vi "CODMn流程.vi"   [LabVIEW 2016]
types:
  T1 = enum16{"步骤1", "步骤2", "步骤3", "步骤4", "步骤5", "步骤6", "步骤7", "步骤8", "步骤9", "步骤10"}
  T2 = enum32{"Bad", "Idle", "Run top level", "Running"}
  T3 = cluster{"系统时间":timestamp, "工作状态":u16, "测量模式":u16, "告警代码":enum16{"无告警", "缺试剂告警", "缺水样告警", "缺蒸馏水告警", "缺标液告警", "仪表漏液告警", "标定异常告警", "超量程告警", "加热异常", "低试剂预警", "超上限告警", "超下限告警", "仪表内部其他异常", "滴定异常告警", "电极异常告警", "量程切换告警", "参数设置告警", "PH电极电位异常", "电导率电极异常", "浊度光度异常", "溶解氧电极异常", "溶解氧光强异常", "温度异常告警", "PH异常告警", "溶解氧异常告警", "电导率异常告警", "浊度异常告警", "叶绿素异常告警", "藻密度异常告警", "蓝绿藻异常告警", "ORP异常告警", "氨氮异常告警", "清洁刷异常告警", "SD卡异常告警", "蓝牙异常告警", "Wifi异常告警", "流程异常告警"}, "故障代码":enum16{"无故障", "电机故障", "温度故障", "通讯故障", "滴定故障"}, "日志代码":u16, "软件版本":u16, "F0":sgl, "F1":sgl, "F2":sgl, "F3":sgl, "T":sgl, "H":sgl, "id":u16, "flowid":u16, "量程":u16}
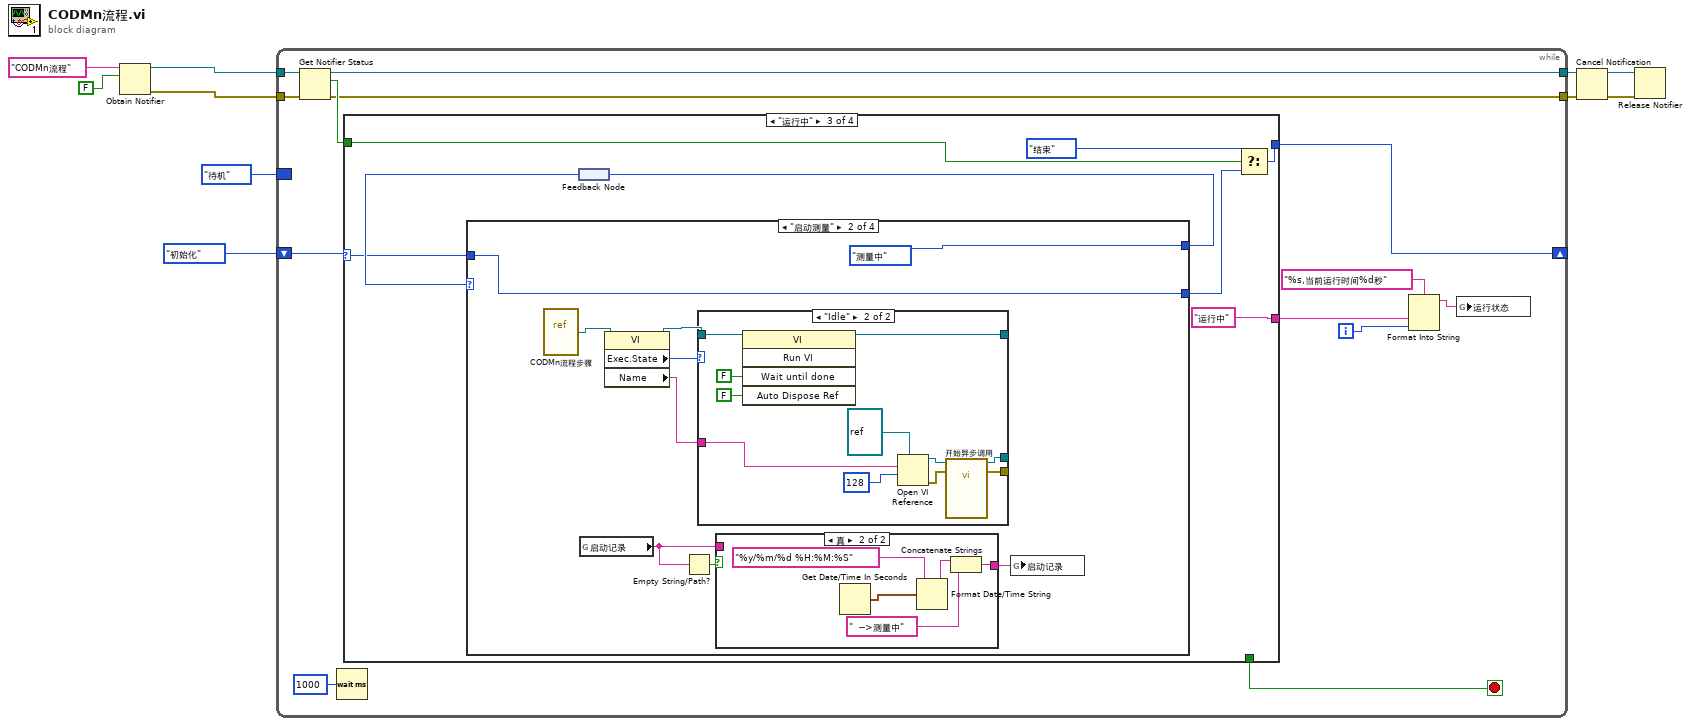
[diagram p0: block diagram]
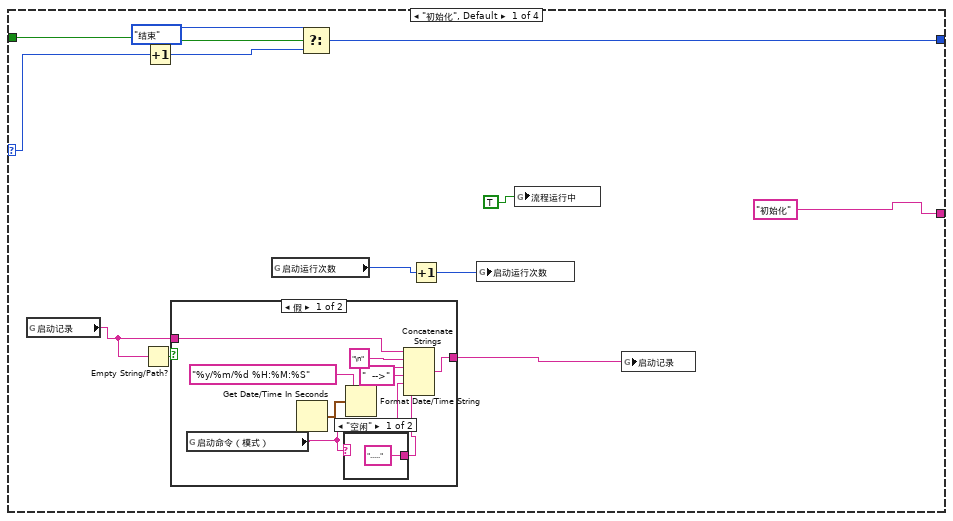
[diagram p2: hidden frame]
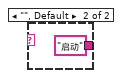
[diagram p3: hidden frame]
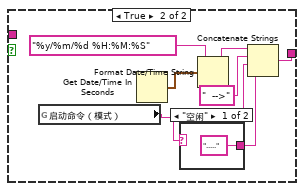
[diagram p4: hidden frame]
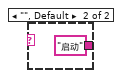
[diagram p5: hidden frame]
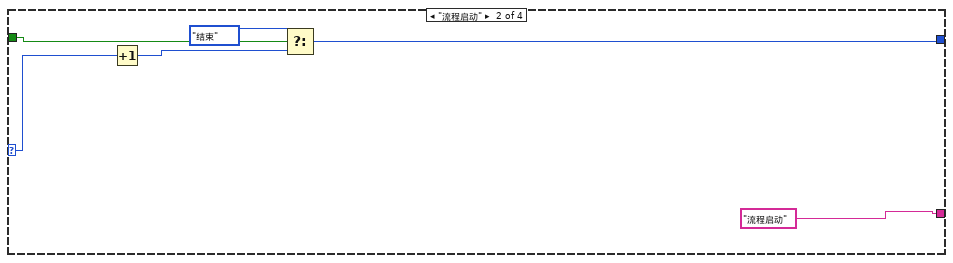
[diagram p6: hidden frame]
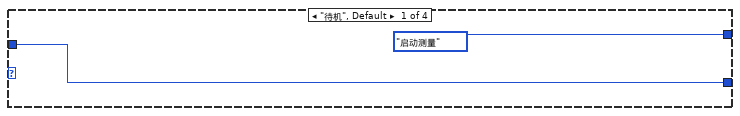
[diagram p7: hidden frame]
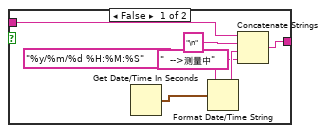
[diagram p8: hidden frame]
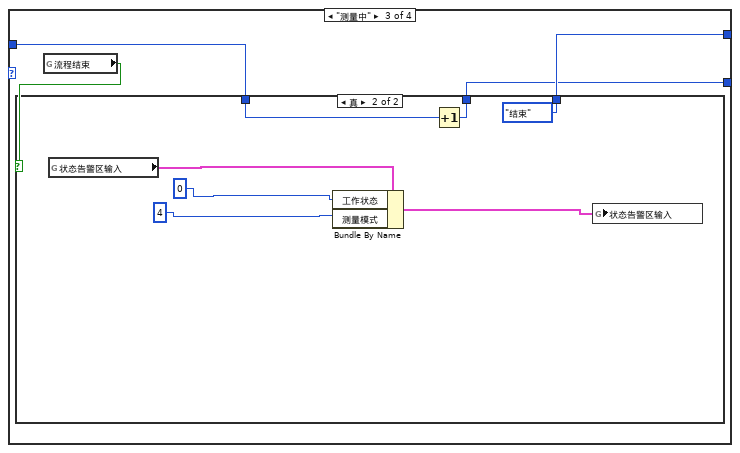
[diagram p10: hidden frame]
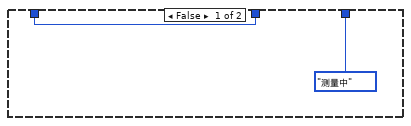
[diagram p11: hidden frame]
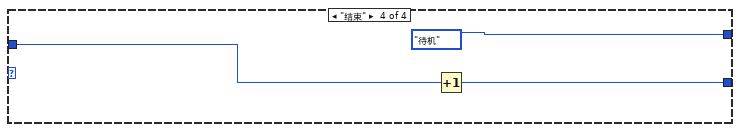
[diagram p12: hidden frame]
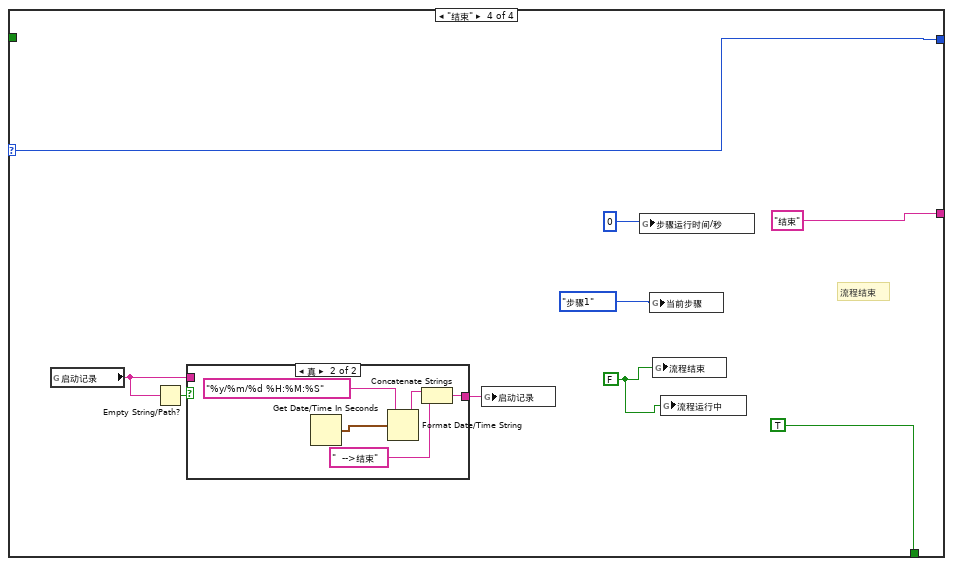
[diagram p13: hidden frame]
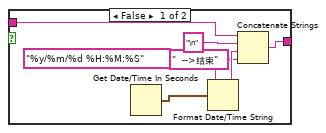
[diagram p14: hidden frame]
diagram:
  n1 = Obtain Notifier(name (unnamed)="CODMn流程" ("名称（未命名）"), notification data type=FALSE) -> (notifier out=w7:refnum<notifier>, error out=w6:errorcluster)  [unwired: 2 in, 1 out]
  n2 = while {
    shift-right: [w20] -> _
    shift-left: enum16{"初始化", "流程启动", "运行中", "结束"}."初始化" ("枚举") -> [w23]
    tunnel: w7 -> [w15]
    tunnel: w6 -> [w14]
    tunnel: [w13] -> w5
    tunnel: [w12] -> w4
    border: enum16{"待机", "启动测量", "测量中", "结束"}."待机" -> [_]
    i -> [w18]
    stop <- w16 stop-if-true
    n3 = Get Notifier Status(notifier=w15, error in (no error)=w14) -> (notifier out=w13:refnum<notifier>, current notification=w21:bool, error out=w12:errorcluster)  [unwired: 2 out]
    n4 = Wait (ms)(milliseconds to wait=u32 1000 ("等待时间（毫秒）")) -> ()  [unwired: 1 out]
    n5 = case shown="\"运行中\"" w23 {
      selector: w23 -> [w33 w58 w64 w127]
      tunnel: [_ _ _ TRUE ("x")] -> w16
      tunnel: w21 -> [w35 w59 w68 _]
      tunnel: [w31 w57 w63 w127] -> w20
      tunnel: ["初始化" ("输入 1") "流程启动" ("输入 1") "运行中" ("输入 1") "结束" ("输入 1")] -> w17
      frame "初始化", Default {
        n6 = global read "CODMn全局.vi" "启动记录"() -> (w24:string)
        n7 = Empty String/Path?(string/path=w24) -> (empty?=w29:bool)
        n8 = Increment(x=w33) -> (x+1=w32:enum16{"初始化", "流程启动", "运行中", "结束"})
        n9 = case shown="假" w29 {
          tunnel: w24 -> [w44 _]
          tunnel: [w39 w50] -> w25
          frame False {
            n10 = global read "CODMn全局.vi" "启动命令（模式）"() -> (w37:string)
            n11 = Get Date/Time In Seconds() -> (seconds since 1Jan1904=w42:timestamp)
            n12 = case shown="\"空闲\"" w37 {
              tunnel: ["....." ("字符串") "启动" ("字符串")] -> w36
              frame "空闲" {
              }
              frame "", Default {
              }
            }
            n13 = Format Date/Time String(time format string (%c)="%y/%m/%d %H:%M:%S" ("时间格式字符串(%c)"), seconds (now)=w42) -> (date/time string=w40:string)  [unwired: 1 in]
            n14 = Concatenate Strings(w44, "\n" ("字符串"), w40, "  -->" ("字符串"), w37, w36) -> (w39:string)
          }
          frame True {
            n15 = global read "CODMn全局.vi" "启动命令（模式）"() -> (w48:string)
            n16 = Get Date/Time In Seconds() -> (seconds since 1Jan1904=w53:timestamp)
            n17 = case shown="\"空闲\"" w48 {
              tunnel: ["....." ("字符串") "启动" ("字符串")] -> w47
              frame "空闲" {
              }
              frame "", Default {
              }
            }
            n18 = Format Date/Time String(time format string (%c)="%y/%m/%d %H:%M:%S" ("时间格式字符串(%c)"), seconds (now)=w53) -> (date/time string=w51:string)  [unwired: 1 in]
            n19 = Concatenate Strings(w51, "  -->" ("字符串"), w48, w47) -> (w50:string)
          }
        }
        n20 = global read "CODMn全局.vi" "启动运行次数"() -> (w27:i32)
        n21 = Select(t=enum16{"初始化", "流程启动", "运行中", "结束"}."结束" ("枚举"), s=w35, f=w32) -> (s? t:f=w31:enum16{"初始化", "流程启动", "运行中", "结束"})
        n22 = Increment(x=w27) -> (x+1=w26:i32)
        n23 = global write "CODMn全局.vi" "启动运行次数"(w26) -> ()
        n24 = global write "CODMn全局.vi" "流程运行中"(TRUE ("流程运行中")) -> ()
        n25 = global write "CODMn全局.vi" "启动记录"(w25) -> ()
      }
      frame "流程启动" {
        n26 = Increment(x=w58) -> (x+1=w60:enum16{"初始化", "流程启动", "运行中", "结束"})
        n27 = Select(t=enum16{"初始化", "流程启动", "运行中", "结束"}."结束" ("枚举"), s=w59, f=w60) -> (s? t:f=w57:enum16{"初始化", "流程启动", "运行中", "结束"})
      }
      frame "运行中" {
        n28 = feedback #1() -> (w67:enum16{"待机", "启动测量", "测量中", "结束"})
        n29 = case shown="\"启动测量\"" w67 {
          tunnel: [enum16{"待机", "启动测量", "测量中", "结束"}."启动测量" enum16{"待机", "启动测量", "测量中", "结束"}."测量中" w108 enum16{"待机", "启动测量", "测量中", "结束"}."待机"] -> w66
          tunnel: [w70 w79 w106 w119] -> w65
          tunnel: w64 -> [w70 w79 w107 w118]
          frame "待机", Default {
          }
          frame "启动测量" {
            n30 = vi-ref "CODMn流程步骤.vi"() -> (w75:refnum<vi>)
            n31 = global read "CODMn全局.vi" "启动记录"() -> (w73:string)
            n32 = property class="VI"(reference=w75) -> (reference out=w76:refnum<vi>, "Exec.State"=w77:T2, "Name"=w78:string)  [unwired: 1 in, 1 out]
            n33 = Empty String/Path?(string/path=w73) -> (empty?=w74:bool)
            n34 = case shown="\"Idle\"" w77 {
              tunnel: w76 -> [w93 w101]
              tunnel: [w93 w102] -> _
              tunnel: w78 -> [_ w100]
              tunnel: [_ w95] -> _
              tunnel: [_ w94] -> _
              frame "Bad", Default {
              }
              frame "Idle" {
                n35 = invoke class="VI" method="Run VI"(reference=w101, "Wait until done"=FALSE ("结束前等待"), "Auto Dispose Ref"=FALSE ("自动销毁引用")) -> (reference out=w102:refnum<vi>)  [unwired: 2 in, 4 out]
                n36 = Open VI Reference(type specifier VI Refnum (for type only)=refnum<vi> refnum ("类型说明符VI引用句柄（仅用于类型）"), vi path=w100, options=128 ("选项")) -> (vi reference=w96:refnum<vi>, error out=w98:errorcluster)  [unwired: 3 in]
                n37 = call-by-ref "开始异步调用"(reference=w96, error in=w98) -> (reference out=w95:refnum<vi>, error out=w94:errorcluster)  [unwired: 12 in]
              }
            }
            n38 = case shown="真" w74 {
              tunnel: w73 -> [w87 _]
              tunnel: [w81 w88] -> w72
              frame False {
                n39 = Get Date/Time In Seconds() -> (seconds since 1Jan1904=w85:timestamp)
                n40 = Format Date/Time String(time format string (%c)="%y/%m/%d %H:%M:%S" ("时间格式字符串(%c)"), seconds (now)=w85) -> (date/time string=w83:string)  [unwired: 1 in]
                n41 = Concatenate Strings(w87, "\n" ("字符串"), w83, "  -->测量中" ("字符串")) -> (w81:string)
              }
              frame True {
                n42 = Get Date/Time In Seconds() -> (seconds since 1Jan1904=w92:timestamp)
                n43 = Format Date/Time String(time format string (%c)="%y/%m/%d %H:%M:%S" ("时间格式字符串(%c)"), seconds (now)=w92) -> (date/time string=w90:string)  [unwired: 1 in]
                n44 = Concatenate Strings(w90, "  -->测量中" ("字符串")) -> (w88:string)
              }
            }
            n45 = global write "CODMn全局.vi" "启动记录"(w72) -> ()
          }
          frame "测量中" {
            n46 = global read "CODMn全局.vi" "流程结束"() -> (w105:bool)
            n47 = case shown="真" w105 {
              tunnel: [enum16{"待机", "启动测量", "测量中", "结束"}."测量中" enum16{"待机", "启动测量", "测量中", "结束"}."结束"] -> w108
              tunnel: w107 -> [w109 w116]
              tunnel: [w109 w115] -> w106
              frame False {
              }
              frame True {
                n48 = global read "CODMn全局.vi" "状态告警区输入"() -> (w112:T3)
                n49 = Bundle By Name(cluster=w112, "工作状态"=u16 0, "测量模式"=u16 4) -> (w111:T3)
                n50 = Increment(x=w116) -> (x+1=w115:enum16{"初始化", "流程启动", "运行中", "结束"})
                n51 = global write "CODMn全局.vi" "状态告警区输入"(w111) -> ()
              }
            }
          }
          frame "结束" {
            n52 = Increment(x=w118) -> (x+1=w119:enum16{"初始化", "流程启动", "运行中", "结束"})
          }
        }
        n53 = feedback-in #1(w66) -> ()
        n54 = Select(t=enum16{"初始化", "流程启动", "运行中", "结束"}."结束" ("枚举"), s=w68, f=w65) -> (s? t:f=w63:enum16{"初始化", "流程启动", "运行中", "结束"})
      }
      frame "结束" {
        w121 = FALSE ("流程结束")
        # "流程结束"
        n55 = global read "CODMn全局.vi" "启动记录"() -> (w125:string)
        n56 = Empty String/Path?(string/path=w125) -> (empty?=w126:bool)
        n57 = case shown="真" w126 {
          tunnel: w125 -> [w136 _]
          tunnel: [w130 w137] -> w122
          frame False {
            n58 = Get Date/Time In Seconds() -> (seconds since 1Jan1904=w134:timestamp)
            n59 = Format Date/Time String(time format string (%c)="%y/%m/%d %H:%M:%S" ("时间格式字符串(%c)"), seconds (now)=w134) -> (date/time string=w132:string)  [unwired: 1 in]
            n60 = Concatenate Strings(w136, "\n" ("字符串"), w132, "  -->结束" ("字符串")) -> (w130:string)
          }
          frame True {
            n61 = Get Date/Time In Seconds() -> (seconds since 1Jan1904=w141:timestamp)
            n62 = Format Date/Time String(time format string (%c)="%y/%m/%d %H:%M:%S" ("时间格式字符串(%c)"), seconds (now)=w141) -> (date/time string=w139:string)  [unwired: 1 in]
            n63 = Concatenate Strings(w139, "  -->结束" ("字符串")) -> (w137:string)
          }
        }
        n64 = global write "CODMn全局.vi" "启动记录"(w122) -> ()
        n65 = global write "CODMn全局.vi" "步骤运行时间/秒"(0 ("运行时间/秒")) -> ()
        n66 = global write "CODMn全局.vi" "当前步骤"(T1."步骤1" ("当前步骤 2")) -> ()
        n67 = global write "CODMn全局.vi" "流程结束"(w121) -> ()
        n68 = global write "CODMn全局.vi" "流程运行中"(w121) -> ()
      }
    }
    n69 = Format Into String(format string="%s,当前运行时间%d秒" ("格式字符串"), w17, w18) -> (resulting string=w11:string)  [unwired: 2 in, 1 out]
    n70 = global write "CODMn全局.vi" "运行状态"(w11) -> ()
  }
  n71 = Cancel Notification(0:w5, 3:w4) -> (8:w3:refnum<notifier>, 11:w2:errorcluster)  [unwired: 1 out]
  n72 = Release Notifier(notifier=w3, error in (no error)=w2) -> ()  [unwired: 1 in, 3 out]
